vi "SPI Is Busy.vi"(8 "error in (no error)":errorcluster, 10 "state":bool, 11 "handle":u32) -> (0 "error out":errorcluster, 1 "function return":u32, 2 "state out":bool, 3 "handle out":u32)   [LabVIEW 2016, in "libMPSSE-SPI.lvlib"]
doc: "FTDI_API FT_STATUS SPI_IsBusy(FT_HANDLE handle, bool *state);"
uses:
  libMPSSE-SPI.lvlib
  libMPSSE.dll
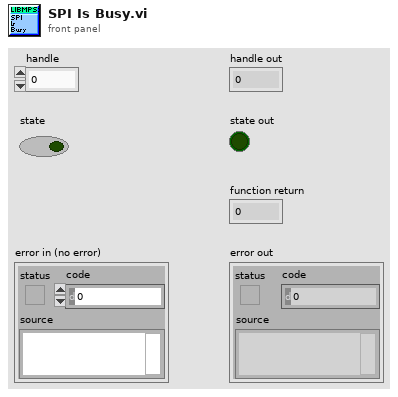
[diagram p1: front panel]
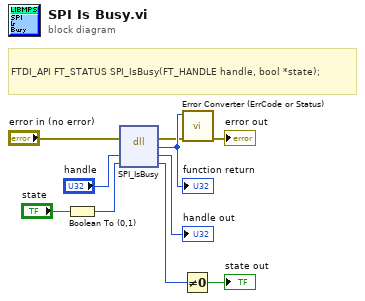
[diagram p0: block diagram]
diagram:
  # "FTDI_API FT_STATUS SPI_IsBusy(FT_HANDLE handle, bool *state);"
  n1 = Boolean To (0,1)(Boolean="state") -> (0, 1=w6:i16)
  n2 = dll-call lib="C:/Users/inca/Desktop/FTDI/libMPSSE-SPI LabVIEW/libMPSSE.*" fn="SPI_IsBusy"(error in="error in (no error)", "handle"="handle", "state"=w6) -> (error out=w2:errorcluster, w10:u32, "handle"=→"handle out":u32, "state"=w4:u8)  [unwired: 2 in, 1 out]
  "function return" <- w10
  n3 = Not Equal To 0?(x=w4) -> (x != 0?=→"state out":bool)
  n4 = call "Error Converter (ErrCode or Status).vi"("error in (no error)"=w2, "error code"=w10) -> ("error out"=→"error out":errorcluster)  [unwired: 9 in]
